vi "SQLite Open V2.vi"(8 "error in":errorcluster, 11 "File Path":path) -> (0 "error out":errorcluster, 2 "Connected?":bool, 3 "SQLite Connection":refnum<class "Connection.lvclass">)   [LabVIEW 2021, in "EDT SQLite+.lvlib"]
uses:
  <vilib>/drjdpowell/SQLite Library/SQL Connection/Connection.lvclass
  <vilib>/drjdpowell/SQLite Library/SQL Connection/Open (path).vi
  <vilib>/drjdpowell/SQLite Library/SQL Connection/Open (string).vi
  <userlib>/_OpenG.lib/file/file.llb/File Exists - Scalar__ogtk.vi
  <vilib>/AdvancedString/Path To Command Line String.vi
  EDT SQLite+.lvlib
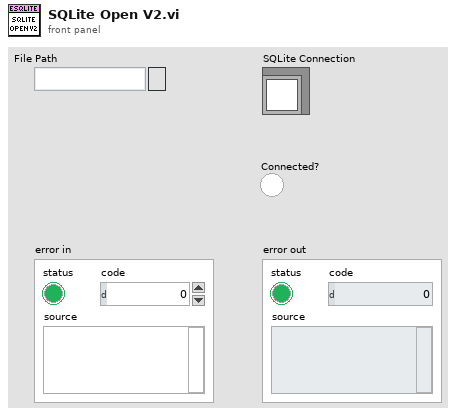
[diagram p1: front panel]
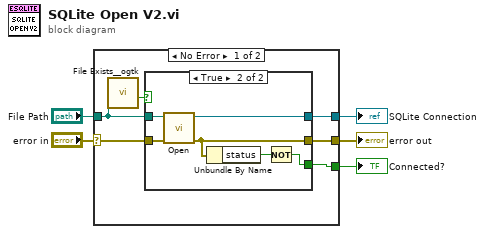
[diagram p0: block diagram]
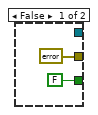
[diagram p2: hidden frame]
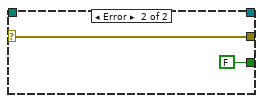
[diagram p3: hidden frame]
diagram:
  n1 = case shown="No Error" "error in" {
    selector: "error in" -> [w9 w21]
    tunnel: [w11 w21] -> w4
    tunnel: "File Path" -> [w8 _]
    tunnel: [w7 _] -> w2
    tunnel: [w6 FALSE] -> w1
    frame No Error {
      n2 = call-poly <userlib>:"File Exists__ogtk.vi"("file path"=w8) -> ("exists"=w10:bool)  [unwired: 6 in, 1 out]
      n3 = case shown="True" w10 {
        tunnel: [errorcluster {"status"=TRUE, "code"=5000, "source"="Failed to open connection"} ("error out") w16] -> w11
        tunnel: w9 -> [_ w19]
        tunnel: w8 -> [_ w18]
        tunnel: [_ w17] -> w7
        tunnel: [FALSE w14] -> w6
        frame False {
        }
        frame True {
          n4 = call-poly <vilib>:"Open.vi"("error in (no error)"=w19, "db file"=w18) -> ("error out"=w16:errorcluster, "SQLite Connection"=w17:refnum<class "Connection.lvclass">)  [unwired: 8 in]
          n5 = Unbundle By Name(w16) -> ("status"=w15:bool)
          n6 = Not(x=w15) -> (.not. x?=w14:bool)
        }
      }
    }
    frame Error {
    }
  }
  "error out" <- w4
  "SQLite Connection" <- w2
  "Connected?" <- w1
